vi "FGV.vi"(7 "Get (F) / Set (T)":bool, 8 "error in (no error)":errorcluster, 11 "data in":T1) -> (0 "error out":errorcluster, 3 "data out":T1)   [LabVIEW 2021, in "XNET-CAN-Signal-Logger.lvlib"]
uses:
  XNET-CAN-Signal-Logger.lvlib
  Typedef/Def-FGV Data Type.ctl
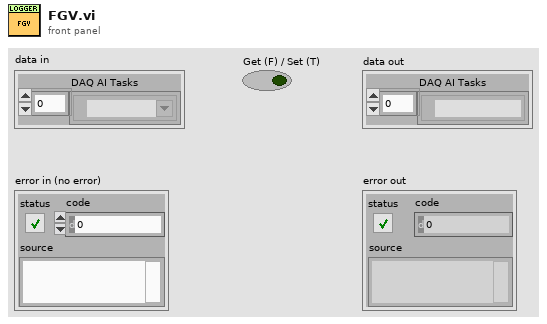
[diagram p1: front panel]
types:
  T1 = typedef "XNET-CAN-Signal-Logger.lvlib/Def-FGV Data Type.ctl" = cluster{"DAQ AI Tasks":refnum<k21>[]}
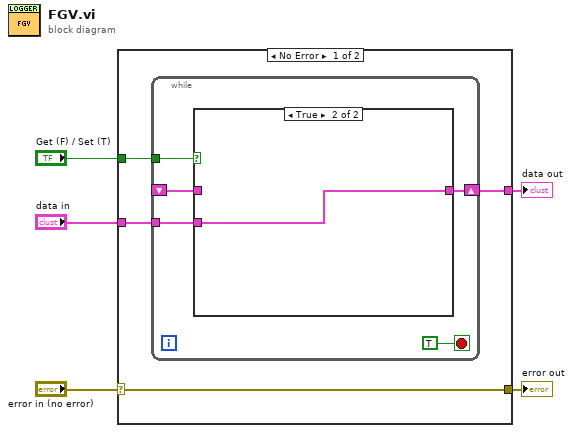
[diagram p0: block diagram]
diagram:
  n1 = case shown="No Error" "error in (no error)" {
    selector: "error in (no error)" -> [w6 w18]
    tunnel: "Get (F) / Set (T)" -> [w9 _]
    tunnel: "data in" -> [w8 w17]
    tunnel: [w7 w17] -> w3
    tunnel: [w6 w18] -> w1
    frame No Error {
      n2 = while {
        tunnel: w9 -> [w13]
        tunnel: w8 -> [w11]
        shift-right: [w12] -> w7
        shift-left: _ -> [w10]
        stop <- TRUE stop-if-true
        n3 = case shown="True" w13 {
          tunnel: [w15 w16] -> w12
          tunnel: w11 -> [_ w16]
          tunnel: w10 -> [w15 _]
          frame False {
          }
          frame True {
          }
        }
      }
    }
    frame Error {
    }
  }
  "data out" <- w3
  "error out" <- w1
